vi "Send RemoveShapeByRef Event.vi"(7 "Auto-Refresh (T)":bool=TRUE, 8 "error in (no error)":errorcluster, 10 "Shape":refnum<data-value>, 11 "Editor Handler in":refnum<class "Image Editor Handler.lvclass">) -> (0 "error out":errorcluster, 3 "Editor Handler out":refnum<class "Image Editor Handler.lvclass">)   [LabVIEW 2015, in "LV Image Editor Framework.lvlib" / "Image Editor Handler.lvclass"]
uses:
  Image Editor Handler.lvclass
  Forms/Shape/Shape.lvclass
  Image Editor Handler.lvclass/Image Editor Handler.ctl
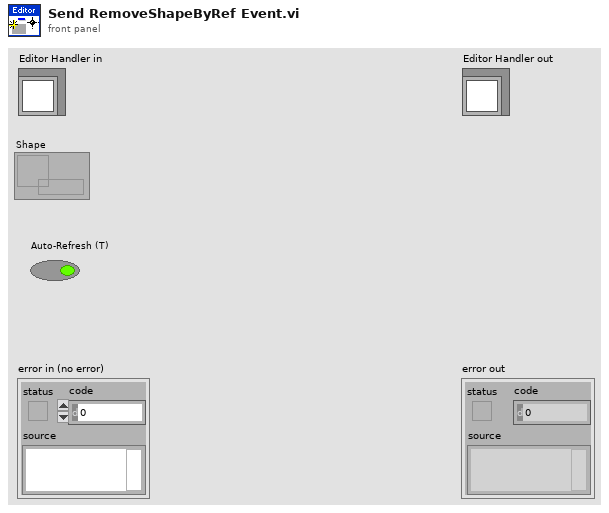
[diagram p1: front panel]
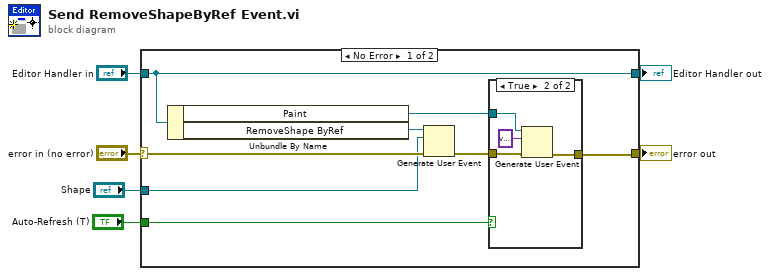
[diagram p0: block diagram]
diagram:
  n1 = case shown="No Error" "error in (no error)" {
    selector: "error in (no error)" -> [w12 w21]
    tunnel: [w9 w21] -> w5
    tunnel: [w14 w20] -> w3
    tunnel: "Editor Handler in" -> [w14 w20]
    tunnel: "Shape" -> [w11 _]
    tunnel: "Auto-Refresh (T)" -> [w8 _]
    frame No Error {
      n2 = Unbundle By Name(w14) -> ("Paint"=w7:refnum<user-event>, "RemoveShape ByRef"=w13:refnum<user-event>)
      n3 = Generate User Event(user event=w13, event data cluster=w11, error in=w12) -> (error out=w10:errorcluster)  [unwired: 1 in, 1 out]
      n4 = case shown="True" w8 {
        tunnel: w10 -> [w15 w19]
        tunnel: [w15 w18] -> w9
        tunnel: w7 -> [_ w17]
        frame False {
        }
        frame True {
          n5 = Generate User Event(user event=w17, event data cluster=variant ("event data"), error in=w19) -> (error out=w18:errorcluster)  [unwired: 1 in, 1 out]
        }
      }
    }
    frame Error {
    }
  }
  "error out" <- w5
  "Editor Handler out" <- w3
